vi "addTwoNumber.vi"(9 "secondNumber":dbl, 10 "firstNumber":dbl, 11 "Model In":refnum<class "Model.lvclass">) -> (3 "Model out":refnum<class "Model.lvclass">)   [LabVIEW 2016, in "Model.lvclass"]
uses:
  Model.lvclass
  Model.lvclass/Model.ctl
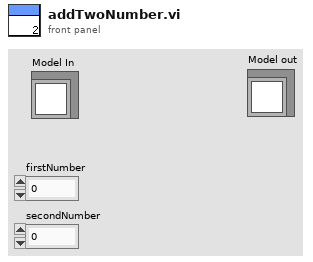
[diagram p1: front panel]
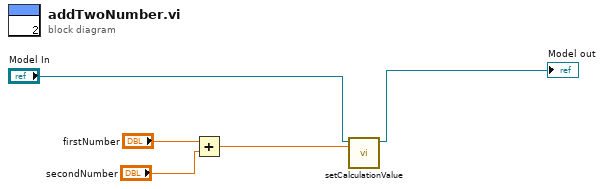
[diagram p0: block diagram]
diagram:
  n1 = Add(x="firstNumber", y="secondNumber") -> (x+y=w3:dbl)
  n2 = call "setCalculationValue.vi"("calculationValue"=w3, "Model in"="Model In") -> ("Model out"=→"Model out":refnum<class "Model.lvclass">)  [unwired: 8 in, 1 out]
